vi "Run Finished.vi"(7 "Run ID":string, 8 "error in":errorcluster, 9 "Result":string, 10 "ts":dbl, 11 "Module ID":i32=-1) -> (0 "error out":errorcluster)   [LabVIEW 2021, in "MQTT Bridge.lvlib"]
doc: "_____\nCreated using DQMH Framework: Event Scripter 7.1.1.1528."
uses:
  MQTT Bridge.lvlib
  Run Finished Argument--cluster.ctl
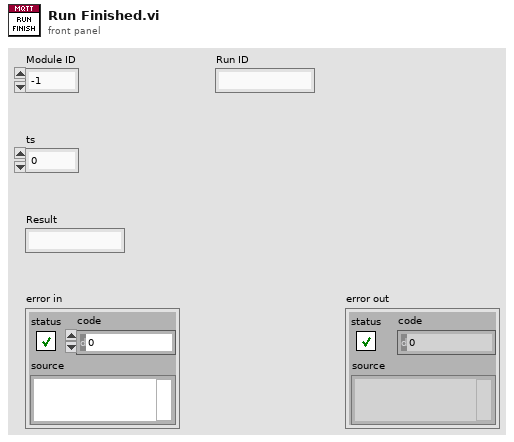
[diagram p1: front panel]
types:
  T1 = typedef "MQTT Bridge.lvlib/Run Finished Argument--cluster.ctl" = cluster{"Module ID":i32, "ts":dbl, "Run ID":string, "Result":string}
  T2 = typedef "MQTT Bridge.lvlib/Request Events--cluster.ctl" = cluster{"Stop Module":refnum<user-event>, "Show Panel":refnum<user-event>, "Hide Panel":refnum<user-event>, "Show Diagram":refnum<user-event>, "Get Module Execution Status":refnum<user-event>, "Connect":refnum<user-event>, "Subscribe":refnum<user-event>, "Update Client Data":refnum<user-event>, "Disconnect":refnum<user-event>, "Check Connection":refnum<user-event>, "Ack Variable Write":refnum<user-event>, "Ack Run Start":refnum<user-event>, "Get Recipe":refnum<user-event>, "Run Finished":refnum<user-event>}
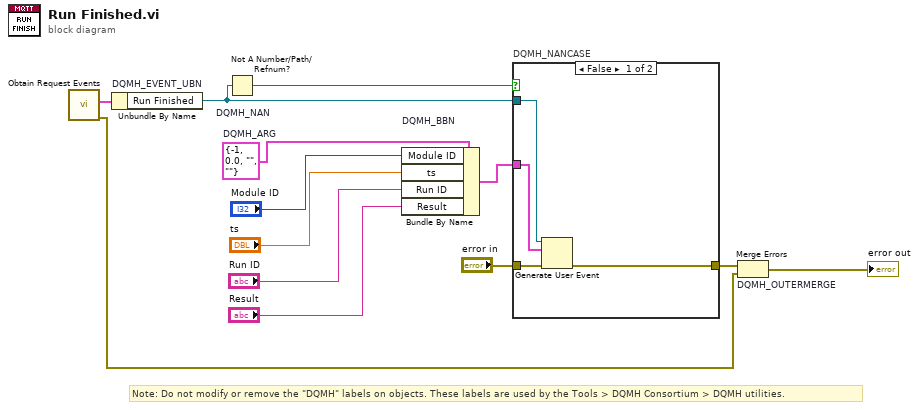
[diagram p0: block diagram]
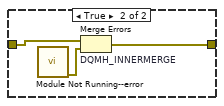
[diagram p2: hidden frame]
diagram:
  w7 = T1 {"Module ID"=-1, "ts"=0.0, "Run ID"="", "Result"=""}  # DQMH_ARG
  # "Note: Do not modify or remove the \"DQMH\" labels on objects. These labels are used by the Tools > DQMH Consortium > DQMH utilities."
  n1 = call "Obtain Request Events.vi"() -> ("error out"=w5:errorcluster, "MQTT Bridge Request Events"=w4:T2)  [unwired: 10 in]
  n2 = Unbundle By Name "DQMH_EVENT_UBN"(w4) -> ("Run Finished"=w9:refnum<user-event>)
  n3 = Not A Number/Path/Refnum? "DQMH_NAN"(number/path/refnum=w9) -> (NaN/Path/Refnum?=w10:bool)
  n4 = Bundle By Name "DQMH_BBN"(cluster=w7, "Module ID"="Module ID", "ts"="ts", "Run ID"="Run ID", "Result"="Result") -> (w11:T1)
  n5 = case "DQMH_NANCASE" shown="False" w10 {
    tunnel: "error in" -> [w17 w20]
    tunnel: [w16 w19] -> w8
    tunnel: w9 -> [w15 _]
    tunnel: w11 -> [w14 _]
    frame False {
      n6 = Generate User Event(user event=w15, event data cluster=w14, error in=w17) -> (error out=w16:errorcluster)  [unwired: 1 in, 1 out]
    }
    frame True {
      n7 = call "Module Not Running--error.vi"() -> ("error out"=w18:errorcluster)  [unwired: 11 in]
      n8 = Merge Errors "DQMH_INNERMERGE"(w20, w18) -> (w19:errorcluster)
    }
  }
  n9 = Merge Errors "DQMH_OUTERMERGE"(w8, w5) -> (→"error out":errorcluster)
